vi "Speed Control Loop.vi"(0 "Loop Gain":dbl=2.0000000000000018 step=0.1, 3 "Enable Speed Control":bool=TRUE, 4 "Speed Feet/Minute":dbl[](array[numeric])=[6.810154191304822, -3.972225965233921e-68], 5 "Right Motor IN":dbl=8.163265306122451, 6 "Left Motor IN":dbl=8.163265306122451) -> (1 "Right Motor OUT":dbl=0.9, 2 "Left Motor OUT":dbl=0.2706222229635261)   [LabVIEW 2012]
uses:
  Robot Global Data.vi
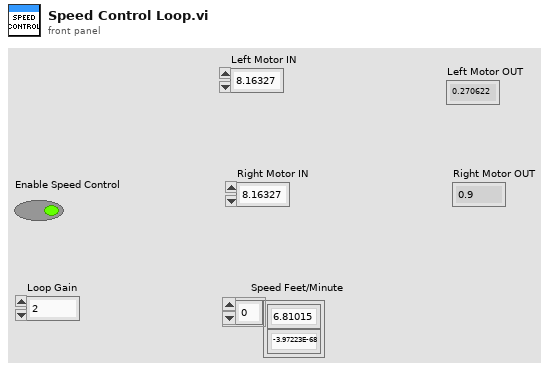
[diagram p1: front panel]
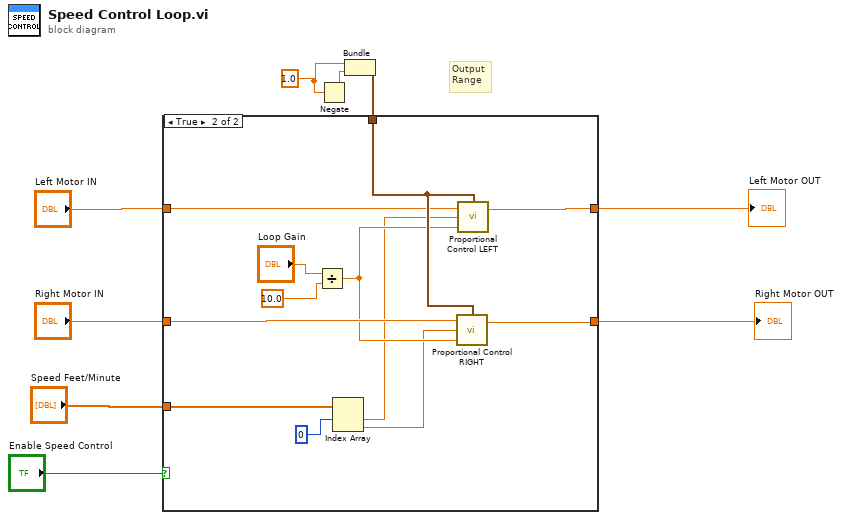
[diagram p0: block diagram]
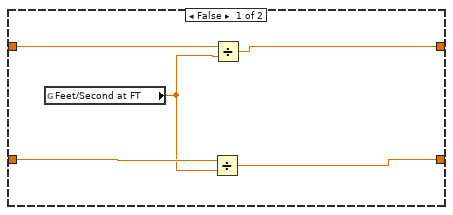
[diagram p2: hidden frame]
diagram:
  w3 = 1.0 ("Max")
  # "Output\nRange"
  n1 = Negate(x=w3) -> (-x=w4:dbl)
  n2 = Bundle("Max"=w3, w4) -> (w2:cluster{"Max":dbl, dbl})  [unwired: 1 in]
  n3 = case shown="True" "Enable Speed Control" {
    tunnel: [w13 w20] -> w8
    tunnel: "Left Motor IN" -> [w14 w18]
    tunnel: "Right Motor IN" -> [w11 w22]
    tunnel: [w12 w21] -> w6
    tunnel: w2 -> [_ w23]
    tunnel: "Speed Feet/Minute" -> [_ w15]
    frame False {
      n4 = global read "Robot Global Data.vi" "Feet/Second at FT"() -> (w10:dbl)
      n5 = Divide(x=w11, y=w10) -> (x/y=w12:dbl)
      n6 = Divide(x=w14, y=w10) -> (x/y=w13:dbl)
    }
    frame True {
      n7 = Divide(x="Loop Gain", y=10.0) -> (x/y=w19:dbl)
      n8 = Index Array(array=w15, index #1=0 ("index")) -> (element #1=w17:dbl, element #2=w16:dbl)  [unwired: 1 in]
      n9 = call "Proportional Control RIGHT.vi"("output range"=w23, "Gain"=w19, "process variable"=w16, "setpoint"=w22) -> ("output"=w21:dbl)  [unwired: 1 out]
      n10 = call "Proportional Control LEFT.vi"("output range"=w23, "Gain"=w19, "process variable"=w17, "setpoint"=w18) -> ("output"=w20:dbl)  [unwired: 1 out]
    }
  }
  "Left Motor OUT" <- w8
  "Right Motor OUT" <- w6
